vi "Pre-Process.vi"(8 "error in":errorcluster, 9 "Actual X position":dbl, 10 "New Data Points":T1, 11 "Scan Driver.lvclass in":refnum<class "Scan Driver.lvclass">) -> (0 "error out":errorcluster, 1 "Secondary Graph":T4, 2 "Primary Graph":T4, 3 "Scan Driver.lvclass out":refnum<class "Scan Driver.lvclass">)   [LabVIEW 2009, in "Scan Driver.lvclass"]
doc: "(Deprecated) Given a new data point, generate one or more auxilliary data points from a secondary source, e.g. a modulator Instrument or an internal computation algorithm. Return the updated onscreen scan graphs with the new data points."
uses:
  Scan Driver.lvclass
  Scan Graph.ctl
  Instruments/Utility Classes/Readable/Data Channels.ctl
  Instruments/Utility Classes/Readable/Data Channel.ctl
  Instruments/Utility Classes/Readable/Data Point.ctl
  Scan Driver.lvclass/Scan Driver.ctl
  Scanners/Scanner/Scanner.lvclass
  Instruments/Utility Classes/Readable/Readable.lvclass
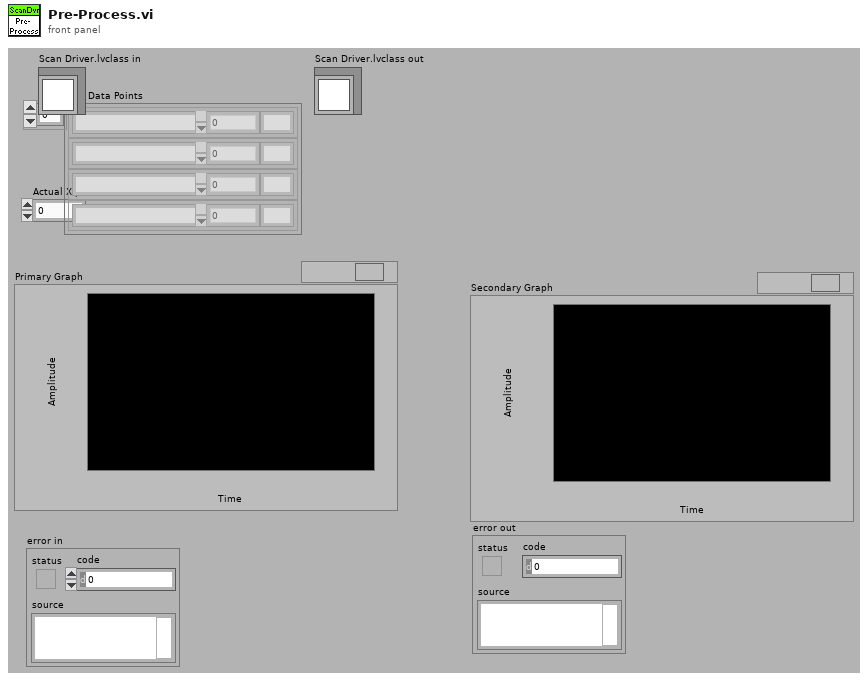
[diagram p1: front panel]
types:
  T1 = typedef "Readable.lvclass/Data Channels.ctl" = T2[]
  T2 = typedef "Readable.lvclass/Data Channel.ctl" = cluster{"Name":string, "Data Point":T3, "Unit":string}
  T3 = typedef "Readable.lvclass/Data Point.ctl" = dbl
  T4 = typedef "Scan Driver.lvclass/Scan Graph.ctl" = cluster{"point array":cluster{"x":dbl, "y":dbl}[]}[]
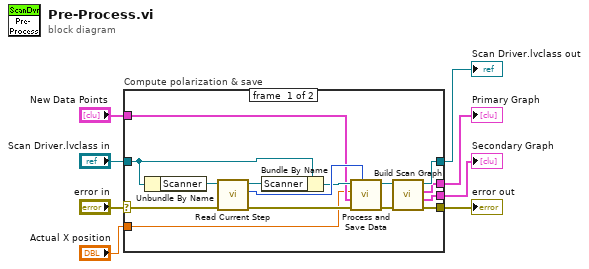
[diagram p0: block diagram]
diagram:
  n1 = case "Compute polarization & save" shown="No Error" "error in" {
    selector: "error in" -> [w12 w25]
    tunnel: "Actual X position" -> [w9 _]
    tunnel: "New Data Points" -> [w10 _]
    tunnel: [w22 _] -> w7
    tunnel: [w21 _] -> w8
    tunnel: [w18 w25] -> w3
    tunnel: [w23 w24] -> w1
    tunnel: "Scan Driver.lvclass in" -> [w17 w24]
    frame #0 {
      n2 = Unbundle By Name(w17) -> ("Scanner"=w16:refnum<class "Scanner.lvclass">)
      n3 = call-dynamic "Read Current Step.vi"("error in (no error)"=w12, "Scanner.lvclass in"=w16) -> ("error out"=w11:errorcluster, "Current Step"=w15:u32, "Scanner.lvclass out"=w13:refnum<class "Scanner.lvclass">)  [unwired: 7 out]
      n4 = Bundle By Name(cluster=w17, "Scanner"=w13) -> (w14:refnum<class "Scan Driver.lvclass">)
      n5 = call-dynamic "Process and Save Data.vi"("step#"=w15, "error in"=w11, "New Data Channels"=w10, "X-Var"=w9, "Scan Driver.lvclass in"=w14) -> ("error out"=w19:errorcluster, "Scan Driver.lvclass out"=w20:refnum<class "Scan Driver.lvclass">)  [unwired: 3 in, 2 out]
      n6 = call-dynamic "Build Scan Graph.vi"("error in"=w19, "Scan Driver in"=w20) -> ("error out"=w18:errorcluster, "Secondary Graph"=w21:T4, "Primary Graph"=w22:T4, "Scan Driver out"=w23:refnum<class "Scan Driver.lvclass">)  [unwired: 4 in, 2 out]
    }
    frame #1 {
    }
  }
  "Secondary Graph" <- w8
  "Primary Graph" <- w7
  "Scan Driver.lvclass out" <- w1
  "error out" <- w3
